vi "trees.vi"() -> ()   [LabVIEW 2009, in "run.lvlib"]
uses:
  run.lvlib
  <vilib>/Utility/miscctls.llb/LVPositionTypeDef.ctl
  Tools/Filing/FileNeologist/FileNeologist.lvclass
panel:
  out "Displayed Items":string[](array[string])
  out "Number of Columns":u32
  out "Active Cell:Position":T1
  in  "Tree":string[](tree)
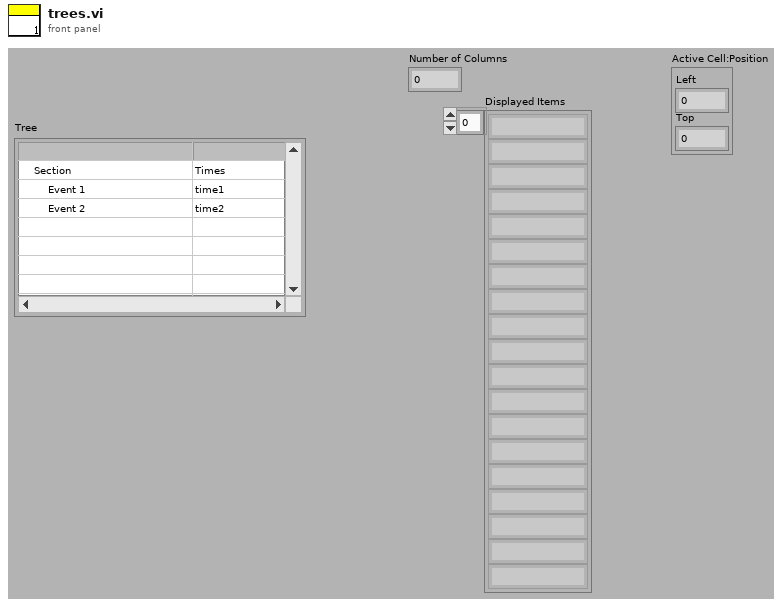
[diagram p1: front panel]
types:
  T1 = typedef "LVPositionTypeDef.ctl" = cluster{"Left":i32, "Top":i32}
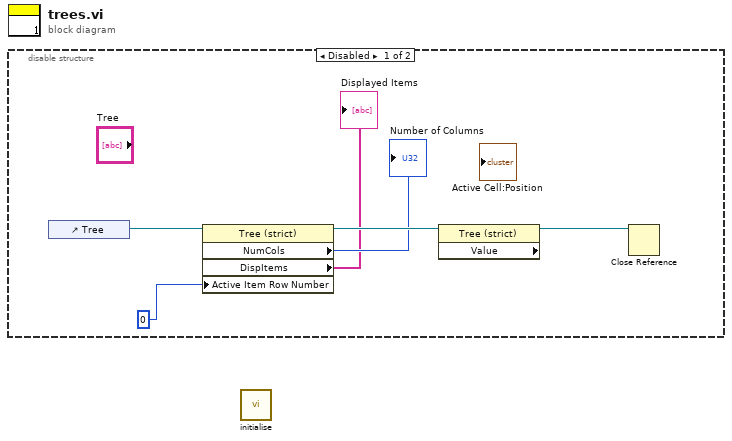
[diagram p0: block diagram]
diagram:
  n1 = disable-structure shown="Disabled" {
    frame #0 {
      n2 = control-ref of="Tree"() -> (w6:refnum<vi>)
      n3 = property class="Tree (strict)"(reference=w6, "Active Item Row Number"=0) -> (reference out=w5:refnum<vi>, "NumCols"=→"Number of Columns":u32, "DispItems"=→"Displayed Items":string[])  [unwired: 1 in, 1 out]
      n4 = property class="Tree (strict)" props=["Value"](reference=w5) -> (reference out=w4:refnum<vi>)  [unwired: 1 in, 2 out]
      n5 = Close Reference(reference=w4) -> ()  [unwired: 1 in, 1 out]
    }
    frame #1 {
    }
  }
  n6 = call "initialise.vi"() -> ()  [unwired: 10 in, 2 out]
